vi "BancadaCalib.vi"() -> ()   [LabVIEW 2014]
uses:
  <vilib>/Analysis/baseanly.llb/Mean (DBL).vi
  <vilib>/Analysis/NI_AALBase.lvlib
panel:
  in  "factor 2":dbl
  out "km/h":dbl format="%#_4f"
  out "Freq":dbl
  out "RPM":dbl format="%#_4f"
  out "input lc (V)":dbl
  out "input tcB (V)":dbl
  out "input tcA (V)":dbl
  out "input ref (V)":dbl
  in  "factor":dbl
  out "hot B(mV)":dbl
  out "tc B(mV)":dbl
  out "tempB(degC)":dbl
  out "hot A(mV)":dbl
  out "tc A(mV)":dbl
  out "tempA(degC)":dbl
  out "temp Ref (degC)":dbl
  out "Force (Kgf)":dbl format="%#_4f"
  in  "offset":dbl step=0.01 format="%#_2f"
  in  "stop":bool
  out "Emf(Cold - mV)":dbl
  # "Cold Junction Information"
  # "Thermocouple A"
  # "Thermocouple B"
  # "Load Cell"
  # "RPM"
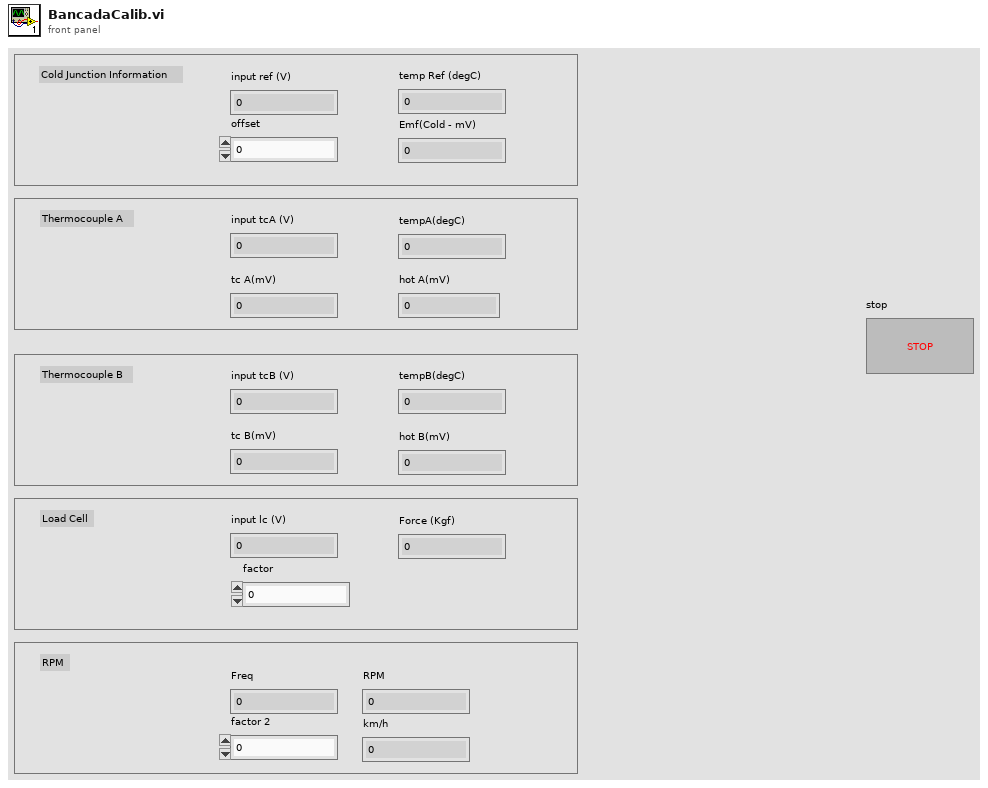
[diagram p1: front panel]
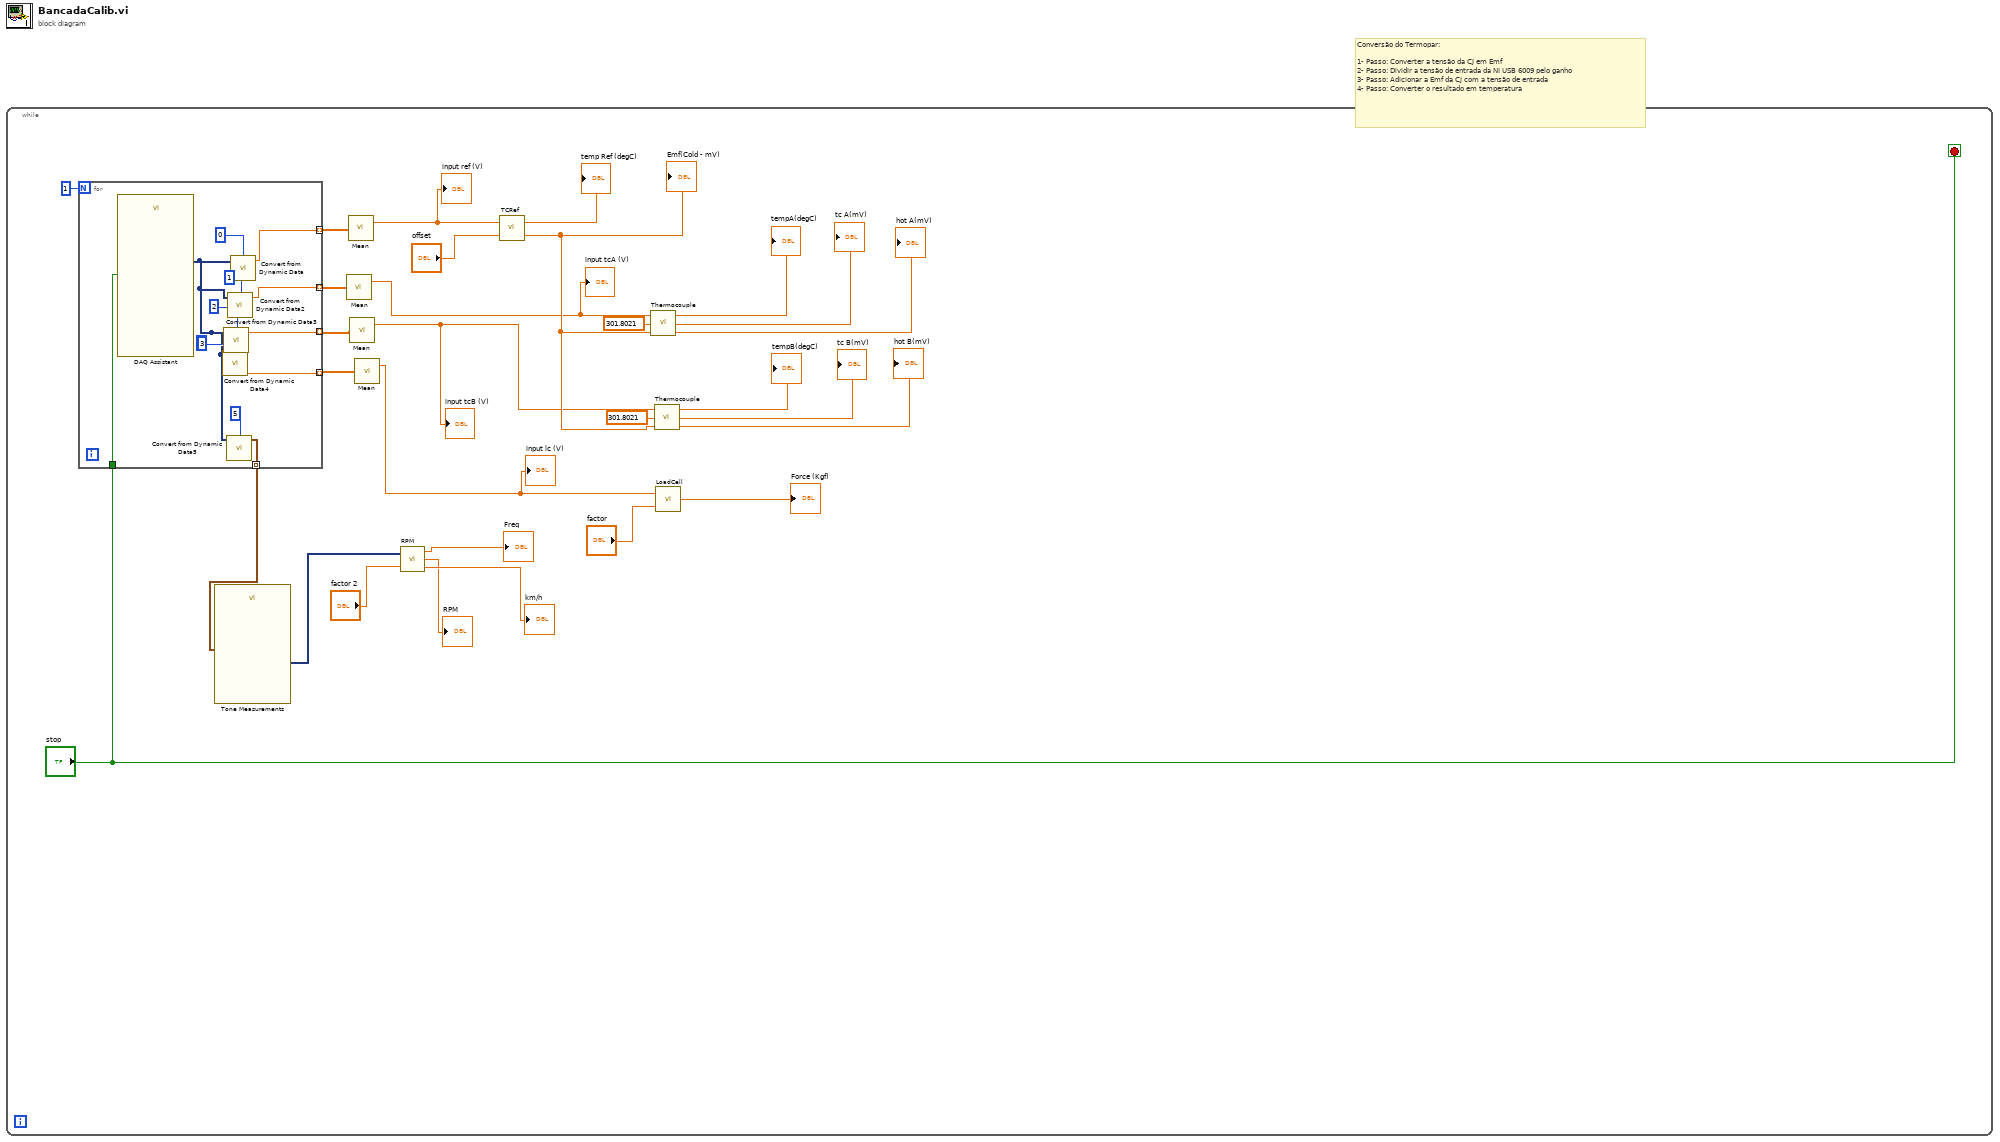
[diagram p0: block diagram]
diagram:
  # "Conversão do Termopar:\n\n1- Passo: Converter a tensão da CJ em Emf\n2- Passo: Dividir a tensão de entrada da NI USB 6009 pelo ganho\n3- Passo: Adicionar a Emf da CJ com a tensão de entrada\n4- Passo: Converter o resultado em temperatura"
  n1 = while {
    stop <- "stop" stop-if-true
    n2 = for {
      N: 1 -> [_]
      tunnel: [w41] -> w28 mode=indexing
      tunnel: [w38] -> w27 mode=indexing
      tunnel: [w36] -> w26 mode=indexing
      tunnel: [w35] -> w25 mode=indexing
      tunnel: "stop" -> [w33]
      tunnel: [w32] -> w1 mode=indexing
      (unwired) 3 ("Channel")
      n3 = call "DAQ Assistant"("stop (F)"=w33) -> ("data"=w30:dynamicdata)  [unwired: 15 in, 3 out]
      n4 = call "Convert from Dynamic Data4"("Dynamic Data Type"=w30, "Channel"=3) -> ("Scalar"=w35:dbl)  [unwired: 2 in]
      n5 = call "Convert from Dynamic Data3"("Dynamic Data Type"=w30, "Channel"=2) -> ("Scalar"=w36:dbl)  [unwired: 2 in]
      n6 = call "Convert from Dynamic Data5"("Dynamic Data Type"=w30, "Channel"=5) -> ("Waveform"=w32:waveform(dbl))  [unwired: 2 in]
      n7 = call "Convert from Dynamic Data2"("Dynamic Data Type"=w30, "Channel"=1) -> ("Scalar"=w38:dbl)  [unwired: 2 in]
      n8 = call "Convert from Dynamic Data"("Dynamic Data Type"=w30, "Channel"=0) -> ("Scalar"=w41:dbl)  [unwired: 2 in]
    }
    n9 = call "Tone Measurements"("Signals"=w1) -> ("Frequency"=w3:dynamicdata)  [unwired: 9 in, 1 out]
    n10 = call-poly <vilib>:"Mean.vi"("X"=w27) -> ("mean"=w10:dbl)  [unwired: 1 out]
    "input tcA (V)" <- w10
    n11 = call-poly <vilib>:"Mean.vi"("X"=w28) -> ("mean"=w11:dbl)  [unwired: 1 out]
    "input ref (V)" <- w11
    n12 = call-poly <vilib>:"Mean.vi"("X"=w26) -> ("mean"=w8:dbl)  [unwired: 1 out]
    "input tcB (V)" <- w8
    n13 = call-poly <vilib>:"Mean.vi"("X"=w25) -> ("mean"=w9:dbl)  [unwired: 1 out]
    "input lc (V)" <- w9
    n14 = call "RPM.vi"("data"=w3, "factor"="factor 2") -> ("Frequency"=→"Freq":dbl, "RPM"=→"RPM":dbl, "km/h"=→"km/h":dbl)
    n15 = call "TCRef.vi"("offset"="offset", "data"=w11) -> ("emf(mV)"=w17:dbl, "temp (degC)"=→"temp Ref (degC)":dbl)
    "Emf(Cold - mV)" <- w17
    n16 = call "Thermocouple.vi"("cj(mV)"=w17, "factor"=301.8021, "data"=w10) -> ("hot(mV)"=→"hot A(mV)":dbl, "tc(mV)"=→"tc A(mV)":dbl, "temp(degC)"=→"tempA(degC)":dbl)
    n17 = call "Thermocouple.vi"("cj(mV)"=w17, "factor"=301.8021, "data"=w8) -> ("hot(mV)"=→"hot B(mV)":dbl, "tc(mV)"=→"tc B(mV)":dbl, "temp(degC)"=→"tempB(degC)":dbl)
    n18 = call "LoadCell.vi"("factor"="factor", "data"=w9) -> ("force (Kgf)"=→"Force (Kgf)":dbl)
  }
